vi "Resistor calculator.vi"() -> ()   [LabVIEW 2011]
panel:
  out "Tolerance String":string
  out "Resistance String":string
  in  "Tolerance":u16(ring)=7 items=["Brown", "Red", "Green", "Blue", "Violet", "Grey", "Gold", "Silver"]
  in  "Multiplier":u16(ring)=2 items=["Black", "Brown", "Red", "Orange", "Yellow", "Green", "Blue", "Violet"]
  in  "Band 3":u16(ring) items=["Black", "Brown", "Red", "Orange", "Yellow", "Green", "Blue", "Violet", "Grey", "White"]
  in  "Band 2":u16(ring)=3 items=["Black", "Brown", "Red", "Orange", "Yellow", "Green", "Blue", "Violet", "Grey", "White"]
  in  "Band 1":u16(ring)=3 items=["Black", "Brown", "Red", "Orange", "Yellow", "Green", "Blue", "Violet", "Grey", "White"]
  out "Resistance":string="33.0k ± 10%"
  in  "Configuration":enum16{"4-Band Code", "5-Band Code"}(ring)=enum."5-Band Code"
  # "Select 4 or 5 band\nconfiguration."
  # "Click colours to match\nthe resistor."
  # "View resistance value."
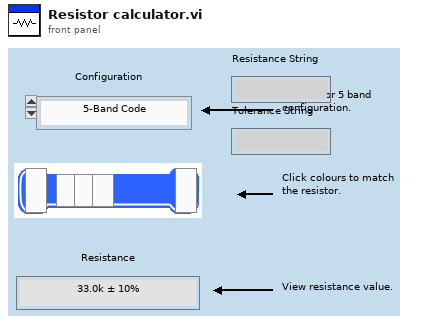
[diagram p1: front panel]
types:
  T1 = enum32{"invalid app kind", "Development System", "Run Time System", "Student Edition", "Embedded LabVIEW", "Evaluation", "Custom"}
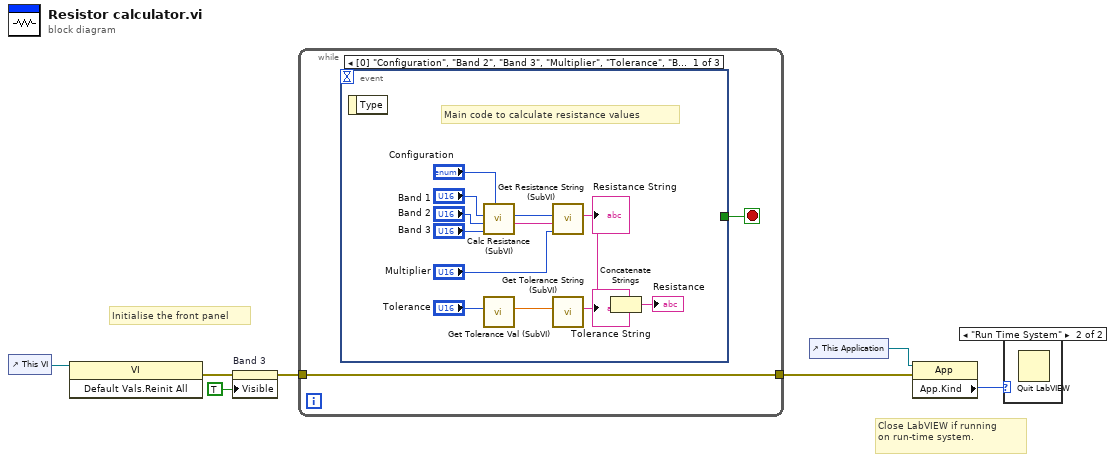
[diagram p0: block diagram]
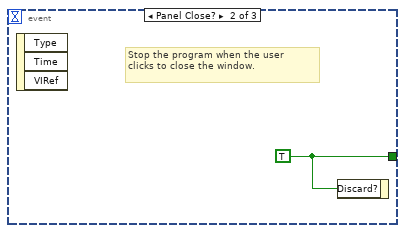
[diagram p3: hidden frame]
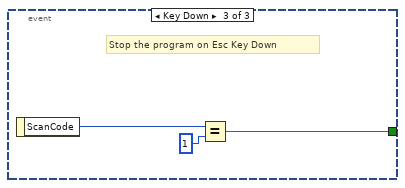
[diagram p4: hidden frame]
diagram:
  # "Close LabVIEW if running\non run-time system."
  # "Initialise the front panel"
  n1 = control-ref of="This VI"() -> (w7:refnum<vi>)
  n2 = invoke class="VI" method="Default Vals.Reinit All"(reference=w7) -> (error out=w5:errorcluster)  [unwired: 2 in, 2 out]
  n3 = property on="Band 3" class="Ring (严格)"(error in=w5, "Visible"=TRUE) -> (error out=w4:errorcluster)  [unwired: 1 in, 1 out]
  n4 = while {
    tunnel: w4 -> [w8]
    tunnel: [w8] -> w1
    stop <- w9 stop-if-true
    n5 = event shown="[0] \"Configuration\", \"Band 2\", \"Band 3\", \"Multiplier\", \"Tolerance\", \"Band 1\": 值改变" {
      selector: _ -> [_ _ _]
      dyn-events: _ -> [_ _ _]
      timeout: _ -> [_ _ _]
      tunnel: [_ w22 w23] -> w9
      event "Configuration", "Band 2", "Band 3", "Multiplier", "Tolerance", "Band 1": Value Change {
        # "Main code to calculate resistance values"
        n6 = event-data() -> ()  [unwired: 1 in, 1 out]
        n7 = call "Calc Resistance (SubVI).vi"("Configuration"="Configuration", "Band 3"="Band 3", "Band 2"="Band 2", "Band 1"="Band 1") -> ("Format String"=w14:string, "Resistance Value"=w15:i32)  [unwired: 5 in, 1 out]
        n8 = call "Get Tolerance Val (SubVI).vi"("Tolerance"="Tolerance") -> ("Tolerance Value"=w11:dbl)  [unwired: 10 in]
        n9 = call "Get Resistance String (SubVI).vi"("Multiplier"="Multiplier", "Format String"=w14, "Resistance Value"=w15) -> ("Resistance String"=w12:string)  [unwired: 8 in]
        "Resistance String" <- w12
        n10 = call "Get Tolerance String (SubVI).vi"("Tolerance Value"=w11) -> ("Tolerance String"=w10:string)  [unwired: 10 in]
        "Tolerance String" <- w10
        n11 = Concatenate Strings(w12, w10) -> (→"Resistance":string)
      }
      event Panel Close? {
        w22 = TRUE ("Discard?")
        # "Stop the program when the user\nclicks to close the window."
        n12 = event-data() -> ()  [unwired: 1 in, 3 out]
        n13 = event-data("Discard?"=w22) -> ()  [unwired: 1 in, 1 out]
      }
      event Key Down {
        # "Stop the program on Esc Key Down"
        n14 = event-data() -> ("ScanCode"=w25:i16)  [unwired: 1 in]
        n15 = Equal?(x=w25, y=i16 1) -> (x = y?=w23:bool)
      }
    }
  }
  n16 = control-ref of="This Application"() -> (w3:refnum<vi>)
  n17 = property class="App"(reference=w3, error in=w1) -> ("App.Kind"=w2:T1)  [unwired: 2 out]
  n18 = case shown="\"Run Time System\"" w2 {
    frame Default {
    }
    frame "Run Time System" {
      n19 = Quit LabVIEW() -> ()  [unwired: 1 in]
    }
  }
